vi "myFreqSymp.vi"(6 "基频":u32=50, 7 "同步频率上限 f_tick_ref":u32=1 min=1 max=50, 8 "响应端口额外频率位移":i8(ring) items=["-2次基波"=-2, "-1次基波"=-1, "无位移"=0, "+1次基波"=1, "+2次基波"=2, "对称-2次基波"=98, "对称-1次基波"=99, "对称"=100, "对称+1次基波"=101, "对称+2次基波"=102], 9 "响应(2号)端口类型":u8(ring) items=["单相", "三相αβ系", "三相同步系", "三相正负序"], 10 "注入(1号)端口类型":u8(ring) items=["单相", "三相αβ系", "三相同步系", "三相正负序"], 11 "freqs in":i32[](array[numeric])) -> (0 "f_mes_max":u32=1, 1 "f_tick_min":u32=1, 3 "freqs, measu, comps":i32[][](array[numeric]))   [LabVIEW 2024]
doc: "测量频率组与耦合频率组的生成，去重与去零"
uses:
  <vilib>/gmath/NI_Gmath.lvlib
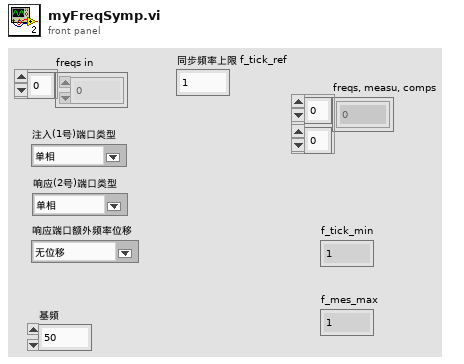
[diagram p1: front panel]
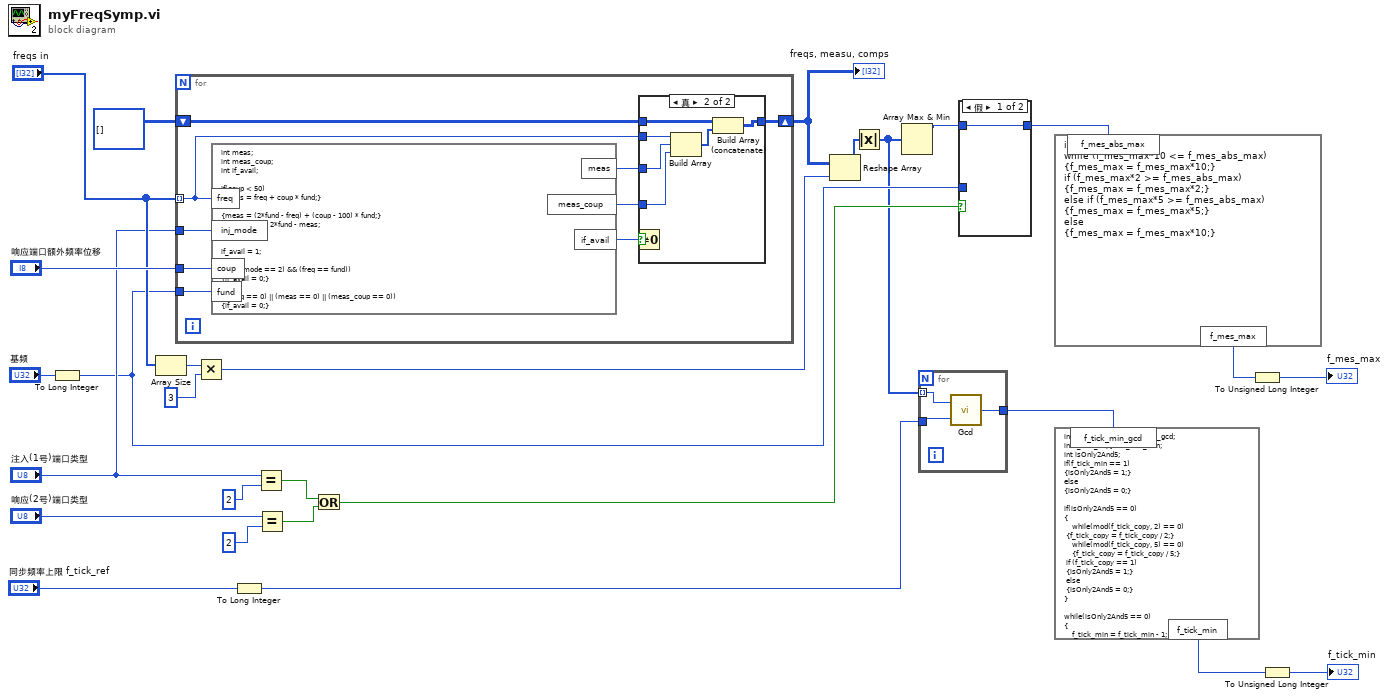
[diagram p0: block diagram]
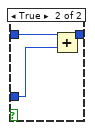
[diagram p2: hidden frame]
diagram:
  n1 = To Long Integer(number="基频") -> (32bit integer=w16:i32)
  n2 = Array Size(array="freqs in") -> (size(s)=w23:i32)
  n3 = for {
    tunnel: "响应端口额外频率位移" -> [w37]
    tunnel: "注入(1号)端口类型" -> [w36]
    tunnel: "freqs in" -> [w28] mode=indexing
    tunnel: w16 -> [w35]
    shift-right: [w31] -> w24
    shift-left: i32[][] [] -> [w32]
    n4 = formula code="int meas;\nint meas_coup;\nint if_avail;\n\nif(coup < 50)\n{meas = freq + coup * fund;}\nelse\n{meas = (2*fund - freq) + (coup - 100) * fund;}\nmeas_coup = 2*fund - meas;\n\n\nif_avail = 1;\n\nif((inj_mode == 2) && (freq == fund))\n{if_avail = 0;}\n\nif((freq == 0) || (meas == 0) || (meas_coup == 0))\n{if_avail = 0;}"("freq"=w28, "coup"=w37, "inj_mode"=w36, "fund"=w35) -> ("meas"=w29:i32, "meas_coup"=w30:i32, "if_avail"=w34:i32)
    n5 = Not Equal To 0?(x=w34) -> (x != 0?=w33:bool)
    n6 = case shown="真" w33 {
      tunnel: w32 -> [w38 w44]
      tunnel: [w38 w43] -> w31
      tunnel: w30 -> [_ w42]
      tunnel: w29 -> [_ w41]
      tunnel: w28 -> [_ w40]
      frame False {
      }
      frame True {
        n7 = Build Array(w40, w41, w42) -> (w39:i32[])
        n8 = Build Array (concatenate)(w44, w39) -> (w43:i32[][])
      }
    }
  }
  "freqs, measu, comps" <- w24
  n9 = Multiply(x=w23, y=3) -> (x*y=w20:i32)
  n10 = To Long Integer(number="同步频率上限 f_tick_ref") -> (32bit integer=w6:i32)
  n11 = Equal?(x="注入(1号)端口类型", y=u8 2) -> (x = y?=w12:bool)
  n12 = Equal?(x="响应(2号)端口类型", y=u8 2) -> (x = y?=w10:bool)
  n13 = Or(x=w12, y=w10) -> (x .or. y?=w11:bool)
  n14 = Reshape Array(w24, w20) -> (w19:i32[])
  n15 = Absolute Value(x=w19) -> (abs(x)=w8:i32[])
  n16 = Array Max & Min(array=w8) -> (max value=w15:i32)  [unwired: 3 out]
  n17 = for {
    tunnel: w8 -> [w47] mode=indexing
    tunnel: w6 -> [w46]
    tunnel: [w45] -> w5
    n18 = call <vilib>:"Gcd.vi"("y"=w46, "x"=w47) -> ("gcd(x,y)"=w45:i32)
  }
  n19 = case shown="假" w11 {
    tunnel: w16 -> [_ w50]
    tunnel: w15 -> [w48 w51]
    tunnel: [w48 w49] -> w9
    frame False {
    }
    frame True {
      n20 = Add(x=w51, y=w50) -> (x+y=w49:i32)
    }
  }
  n21 = formula code="int f_mes_max = 1;\nwhile (f_mes_max*10 <= f_mes_abs_max)\n{f_mes_max = f_mes_max*10;}\nif (f_mes_max*2 >= f_mes_abs_max)\n{f_mes_max = f_mes_max*2;}\nelse if (f_mes_max*5 >= f_mes_abs_max)\n{f_mes_max = f_mes_max*5;}\nelse\n{f_mes_max = f_mes_max*10;}"("f_mes_abs_max"=w9) -> ("f_mes_max"=w3:i32)
  n22 = formula code="int f_tick_min = f_tick_min_gcd;\nint f_tick_copy = f_tick_min;\nint isOnly2And5;\nif(f_tick_min == 1)\n{isOnly2And5 = 1;}\nelse\n{isOnly2And5 = 0;}\n\nif(isOnly2And5 == 0)\n{\n    while(mod(f_tick_copy, 2) == 0)\n\t{f_tick_copy = f_tick_copy / 2;}\n    while(mod(f_tick_copy, 5) == 0)\n    {f_tick_copy = f_tick_copy / 5;}\n\tif (f_tick_copy == 1)\n\t{isOnly2And5 = 1;}\n\telse\n\t{isOnly2And5 = 0;}\n}\n\nwhile(isOnly2And5 == 0)\n{\n    f_tick_min = f_tick_min - 1;\n\n    isOnly2And5 = (f_tick_min == 1);\n    if(isOnly2And5 == 0)\n\t{\n        f_tick_copy = f_tick_min;\n        while(mod(f_tick_copy, 2) == 0)\n        {f_tick_copy = f_tick_copy / 2;}\n        while(mod(f_tick_copy, 5) == 0)\n        {f_tick_copy = f_tick_copy / 5;}\n        if (f_tick_copy == 1)\n\t\t{isOnly2And5 = 1;}\n\t\telse\n\t\t{isOnly2And5 = 0;}\n\t}\n}"("f_tick_min_gcd"=w5) -> ("f_tick_min"=w4:i32)
  n23 = To Unsigned Long Integer(number=w3) -> (unsigned 32bit integer=→"f_mes_max":u32)
  n24 = To Unsigned Long Integer(number=w4) -> (unsigned 32bit integer=→"f_tick_min":u32)
